vi "数码显示.vi"(1 "ascii码":i8) -> (0 "簇":T1)   [LabVIEW 2015]
doc: "查询ASCII码显示数字"
panel:
  out "分1":bool[][](array[boolean])
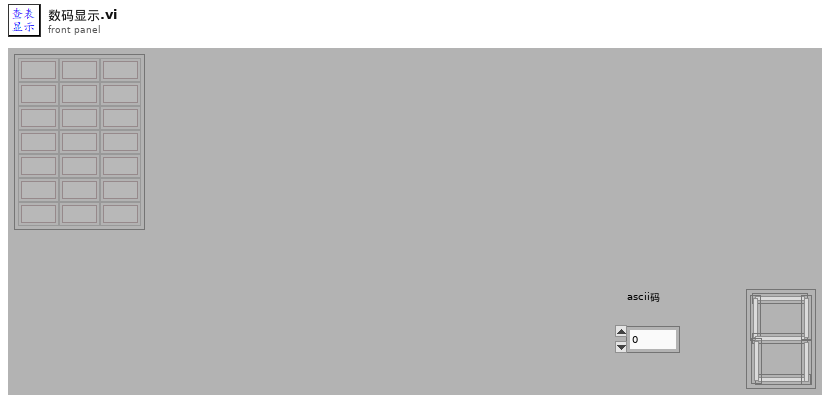
[diagram p1: front panel]
types:
  T1 = cluster{"布尔":bool, "布尔 3":bool, "布尔 2":bool, "布尔 4":bool, "布尔 5":bool, "布尔 6":bool, "布尔 7":bool}
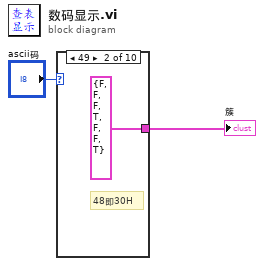
[diagram p0: block diagram]
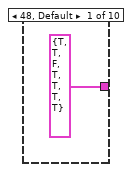
[diagram p2: hidden frame]
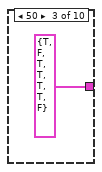
[diagram p3: hidden frame]
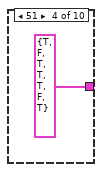
[diagram p4: hidden frame]
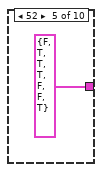
[diagram p5: hidden frame]
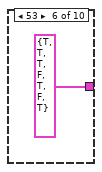
[diagram p6: hidden frame]
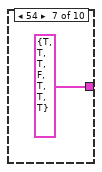
[diagram p7: hidden frame]
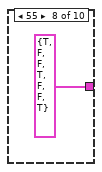
[diagram p8: hidden frame]
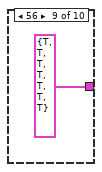
[diagram p9: hidden frame]
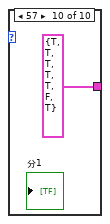
[diagram p10: hidden frame]
diagram:
  n1 = case shown="49" "ascii码" {
    tunnel: [T1 {"布尔"=TRUE, "布尔 3"=TRUE, "布尔 2"=FALSE, "布尔 4"=TRUE, "布尔 5"=TRUE, "布尔 6"=TRUE, "布尔 7"=TRUE} ("簇 3") T1 {"布尔"=FALSE, "布尔 3"=FALSE, "布尔 2"=FALSE, "布尔 4"=TRUE, "布尔 5"=FALSE, "布尔 6"=FALSE, "布尔 7"=TRUE} ("簇 3") T1 {"布尔"=TRUE, "布尔 3"=FALSE, "布尔 2"=TRUE, "布尔 4"=TRUE, "布尔 5"=TRUE, "布尔 6"=TRUE, "布尔 7"=FALSE} ("簇 3") T1 {"布尔"=TRUE, "布尔 3"=FALSE, "布尔 2"=TRUE, "布尔 4"=TRUE, "布尔 5"=TRUE, "布尔 6"=FALSE, "布尔 7"=TRUE} ("簇 3") T1 {"布尔"=FALSE, "布尔 3"=TRUE, "布尔 2"=TRUE, "布尔 4"=TRUE, "布尔 5"=FALSE, "布尔 6"=FALSE, "布尔 7"=TRUE} ("簇 3") T1 {"布尔"=TRUE, "布尔 3"=TRUE, "布尔 2"=TRUE, "布尔 4"=FALSE, "布尔 5"=TRUE, "布尔 6"=FALSE, "布尔 7"=TRUE} ("簇 3") T1 {"布尔"=TRUE, "布尔 3"=TRUE, "布尔 2"=TRUE, "布尔 4"=FALSE, "布尔 5"=TRUE, "布尔 6"=TRUE, "布尔 7"=TRUE} ("簇 3") T1 {"布尔"=TRUE, "布尔 3"=FALSE, "布尔 2"=FALSE, "布尔 4"=TRUE, "布尔 5"=FALSE, "布尔 6"=FALSE, "布尔 7"=TRUE} ("簇 3") T1 {"布尔"=TRUE, "布尔 3"=TRUE, "布尔 2"=TRUE, "布尔 4"=TRUE, "布尔 5"=TRUE, "布尔 6"=TRUE, "布尔 7"=TRUE} ("簇 3") T1 {"布尔"=TRUE, "布尔 3"=TRUE, "布尔 2"=TRUE, "布尔 4"=TRUE, "布尔 5"=TRUE, "布尔 6"=FALSE, "布尔 7"=TRUE} ("簇 3")] -> w1
    frame 48, Default {
    }
    frame 49 {
      # "48即30H"
    }
    frame 50 {
    }
    frame 51 {
    }
    frame 52 {
    }
    frame 53 {
    }
    frame 54 {
    }
    frame 55 {
    }
    frame 56 {
    }
    frame 57 {
    }
  }
  "簇" <- w1
